vi "thermal_optical_camera_V2.vi"() -> ()   [LabVIEW 2025]
panel:
  out "file name out":string
  in  "File Path":string="C:\\Digambar\\Metal_thin_wall\\Optical_images\\Optical_images"
  in  "Stop (F)":bool
  in  "Acquisition Control:\nExposure Time [100, 3E7]":dbl=999.0 caption="Acquisition Control::Exposure Time" min=100.0 max=29999995.0
  in  "Analog Control:\nGain [0, 27]":dbl caption="Analog Control::Gain" min=0.0 max=27.045663671679687
  in  "Analog Control:\nBlack Level [-5, 10]":dbl caption="Analog Control::Black Level" min=-5.0000011920928955 max=10.000002384185791
  in  "Analog Control:\nGamma [0.25, 4.00]":dbl=0.800048828125 caption="Analog Control::Gamma" min=0.25 max=4.0 step=0.05
  out "Optical camera":T1(plugin-control)
  in  "optical capture interval (s)":dbl
  in  "thermal capture interval (s)":dbl
  out "Thermal camera":T1(plugin-control)
  out "IP address":string
  out "Output":string
  in  "Flag Button":bool
  in  "Stop Recording":bool
  in  "Stop Preview":bool
  in  "Focus":dbl(slide) scale=0.0..100.0
  in  "Record":bool
  # "Destination for Optical Images:"
  # "change folder names each time you run,\nso it saves data sets in dedicated folders:\nfolder1\nfolder2\nfolder3\netc..."
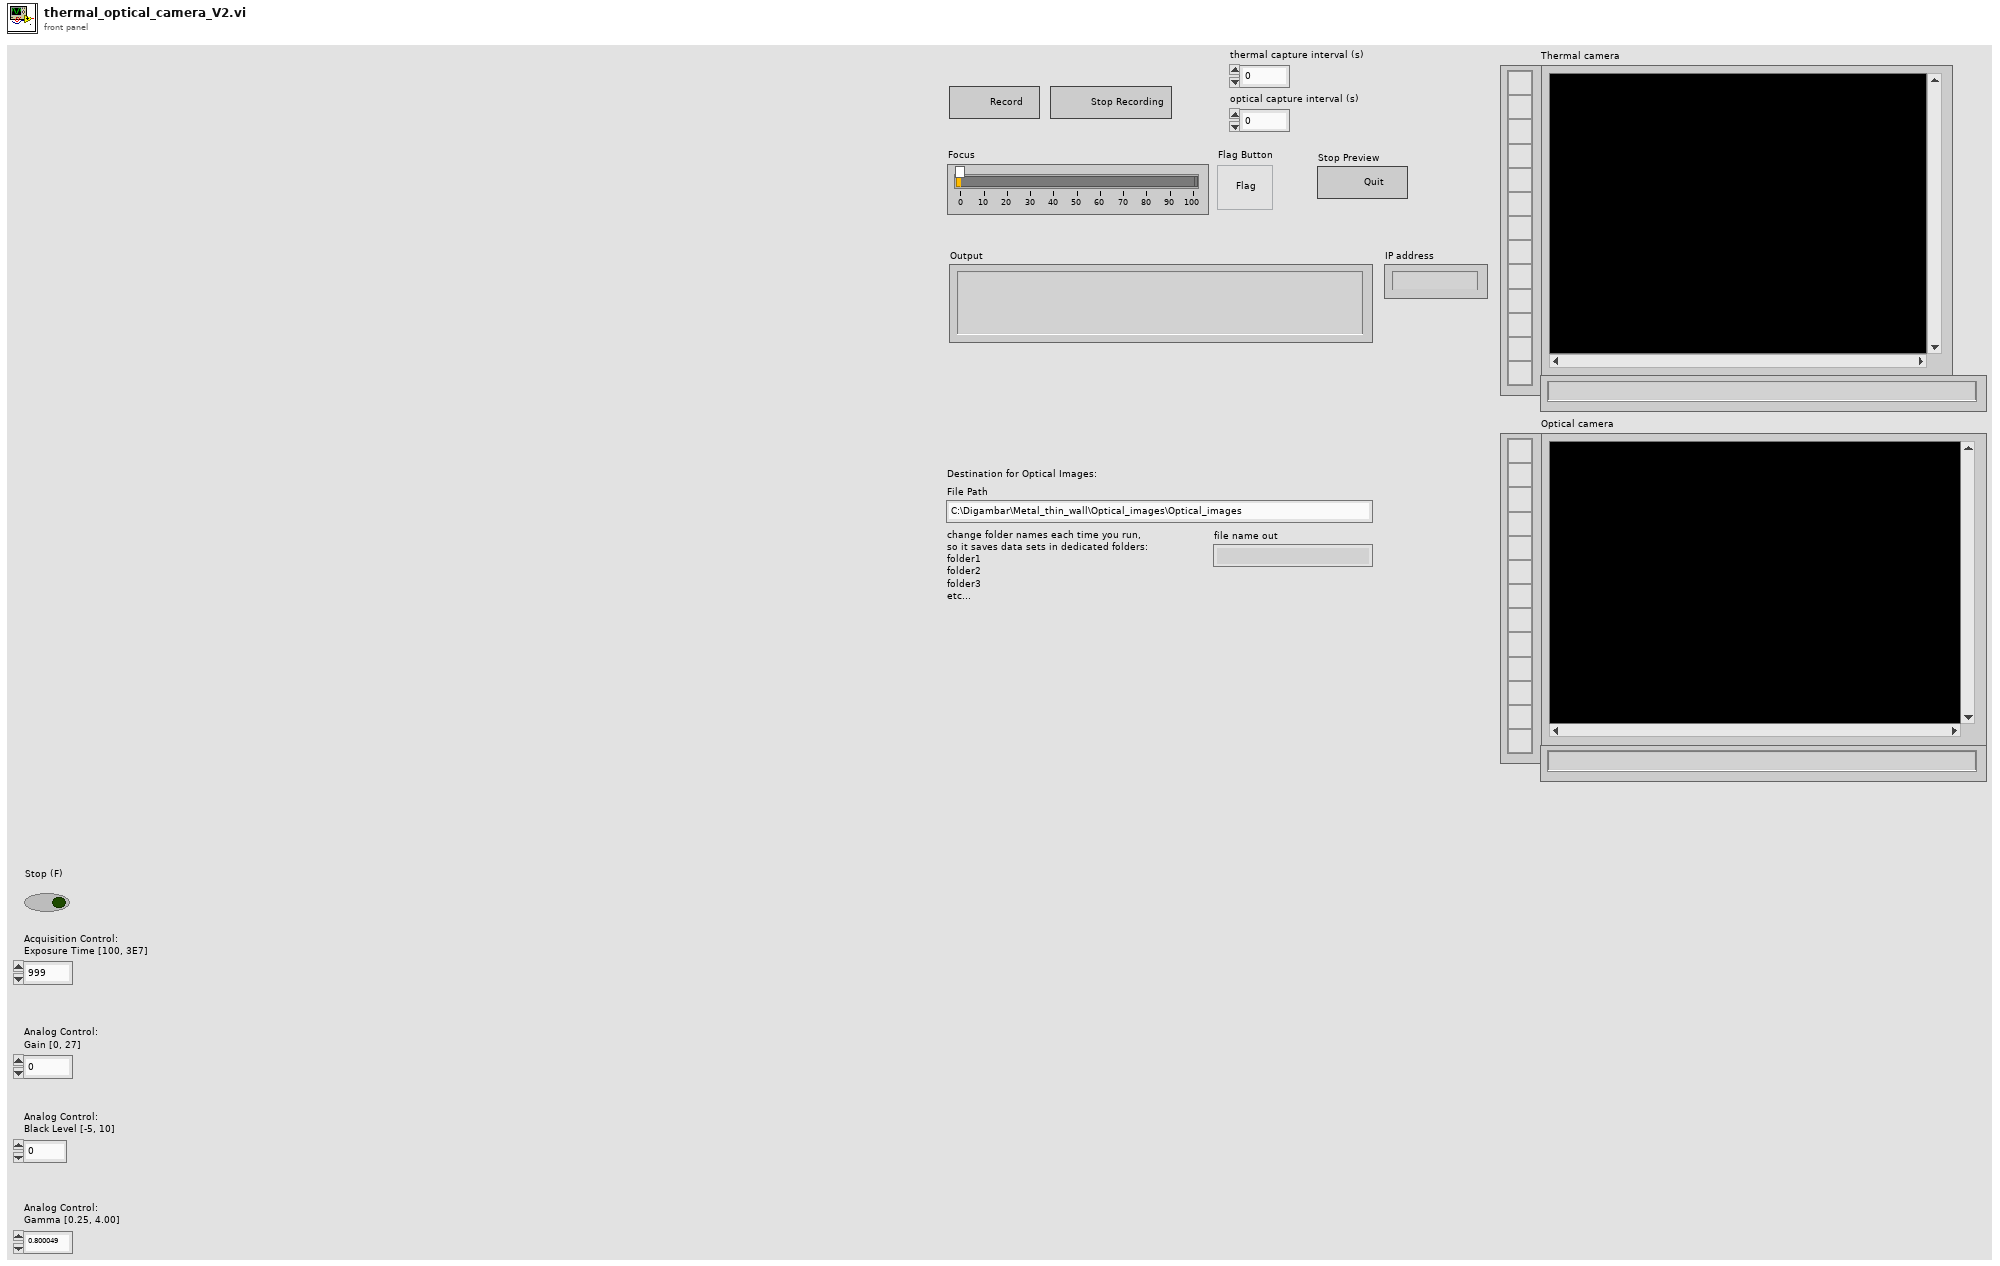
[diagram p1: front panel]
types:
  T1 = typedef "IMAQ Image.ctl" = refnum<image>
  T2 = enum16{"open", "replace", "create", "open or create", "replace or create", "replace or create with confirmation"}
  T3 = enum16{"big-endian, network order", "native, host order", "little-endian"}
  T4 = enum16{"Standard", "Buffered", "CRLF", "Immediate"}
  T5 = typedef "Image Type" = u32
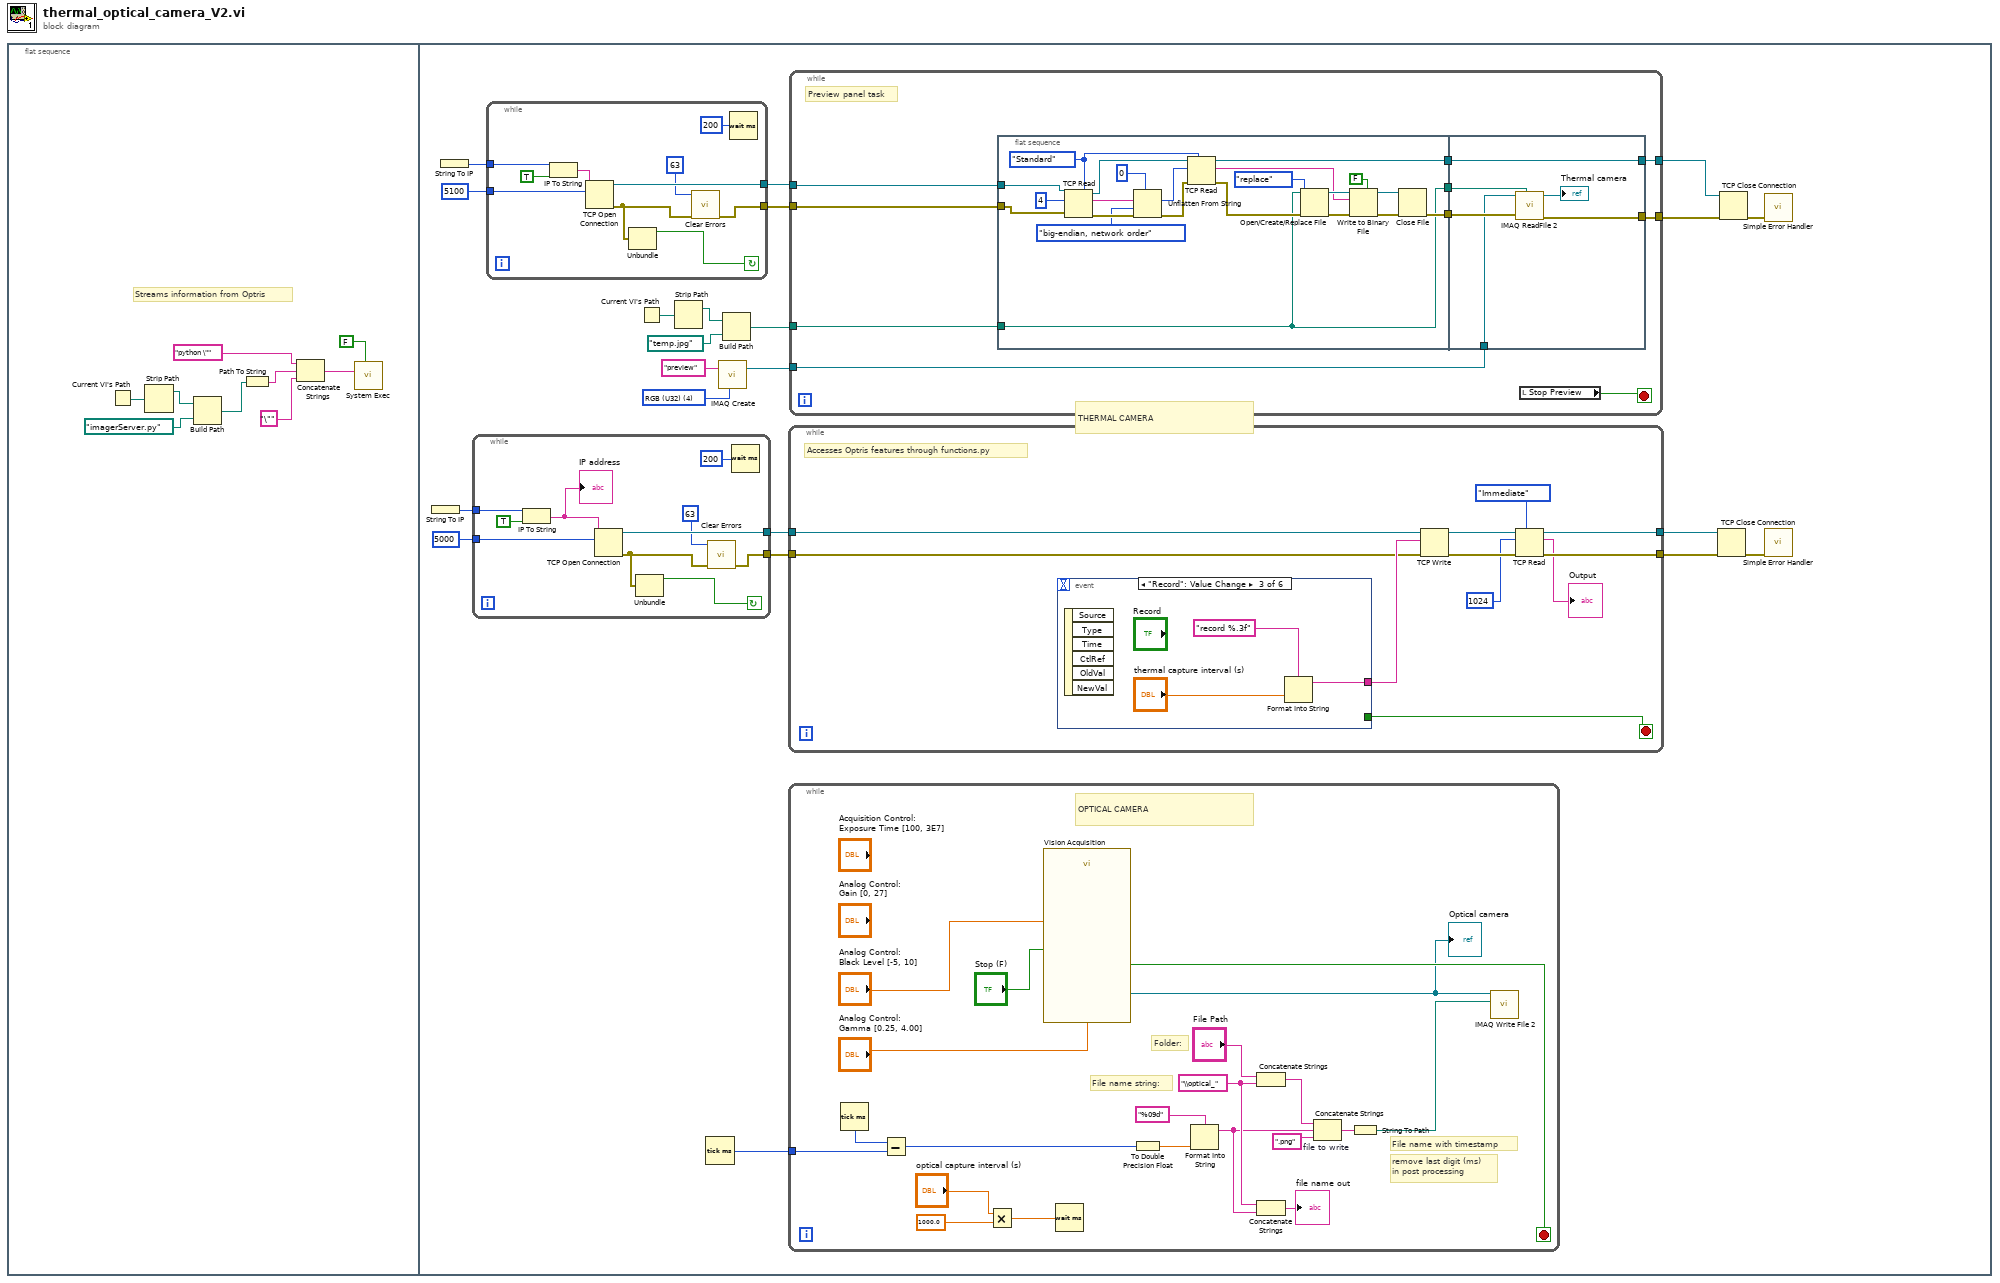
[diagram p0: block diagram]
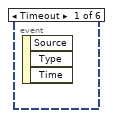
[diagram p2: hidden frame]
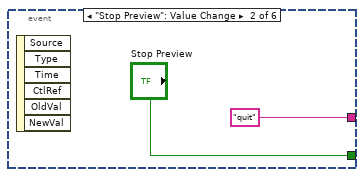
[diagram p3: hidden frame]
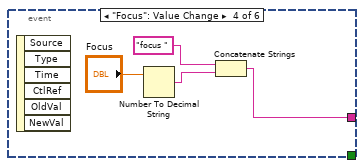
[diagram p4: hidden frame]
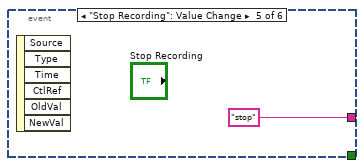
[diagram p5: hidden frame]
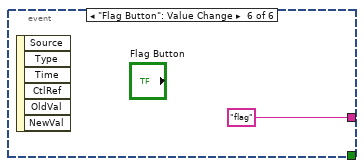
[diagram p6: hidden frame]
diagram:
  n1 = flat-sequence {
    frame #0 {
      # "Streams information from Optris"
      n2 = Current VI's Path() -> (path=w4:path)
      n3 = Strip Path(path=w4) -> (stripped path=w5:path)  [unwired: 1 out]
      n4 = Build Path(base path=w5, name or relative path=path "imagerServer.py") -> (appended path=w2:path)
      n5 = Path To String(path=w2) -> (string=w8:string)
      n6 = Concatenate Strings("python \"" ("string"), w8, "\"" ("string")) -> (w7:string)
      n7 = call <vilib>:"System Exec.vi"("wait until completion? (T)"=FALSE, "command line"=w7) -> ()  [unwired: 6 in, 4 out]
    }
    frame #1 {
      w19 = T5 4 items=["Grayscale (U8)", "Grayscale (I16)", "Grayscale (SGL)", "Complex (CSG)", "RGB (U32)", "HSL (U32)", "RGB (U64)", "Grayscale (U16)"] ("Image Type")
      # "THERMAL CAMERA"
      n8 = String To IP() -> (0:w16:u32)  [unwired: 1 in]
      n9 = String To IP() -> (0:w14:u32)  [unwired: 1 in]
      n10 = while {
        tunnel: [w66] -> w18
        tunnel: [w72] -> w17
        tunnel: w16 -> [w70]
        tunnel: u16 5000 ("remote port or service name") -> [w68]
        stop <- w63 continue-if-true
        n11 = IP To String(1:TRUE ("dot notation? (F)"), 2:w70) -> (0:w71:string)
        "IP address" <- w71
        n12 = TCP Open Connection(address=w71, remote port or service name=w68) -> (connection ID=w72:refnum<k5>, error out=w67:errorcluster)  [unwired: 3 in]
        n13 = Unbundle(w67) -> ("status"=w63:bool)  [unwired: 2 out]
        n14 = call <vilib>:"Clear Errors.vi"("error in (no error)"=w67, "specific error code to clear (0: all)"=63) -> ("error out"=w66:errorcluster)  [unwired: 4 in, 1 out]
        n15 = Wait (ms)(milliseconds to wait=u32 200) -> ()  [unwired: 1 out]
      }
      n16 = while {
        tunnel: w14 -> [w62]
        tunnel: [w56] -> w13
        tunnel: [w60] -> w12
        tunnel: u16 5100 ("remote port or service name") -> [w58]
        stop <- w53 continue-if-true
        n17 = IP To String(1:TRUE ("dot notation? (F)"), 2:w62) -> (0:w61:string)
        n18 = TCP Open Connection(address=w61, remote port or service name=w58) -> (connection ID=w60:refnum<k5>, error out=w57:errorcluster)  [unwired: 3 in]
        n19 = Unbundle(w57) -> ("status"=w53:bool)  [unwired: 2 out]
        n20 = call <vilib>:"Clear Errors.vi"("error in (no error)"=w57, "specific error code to clear (0: all)"=63) -> ("error out"=w56:errorcluster)  [unwired: 4 in, 1 out]
        n21 = Wait (ms)(milliseconds to wait=u32 200) -> ()  [unwired: 1 out]
      }
      n22 = Current VI's Path() -> (path=w30:path)
      n23 = Strip Path(path=w30) -> (stripped path=w31:path)  [unwired: 1 out]
      n24 = Tick Count (ms)() -> (millisecond timer value=w10:u32)
      n25 = call "IMAQ Create"("Image Name"="preview", "Image Type"=w19) -> ("New Image"=w26:T1)  [unwired: 3 in, 1 out]
      n26 = Build Path(base path=w31, name or relative path=path "temp.jpg") -> (appended path=w29:path)
      n27 = while {
        tunnel: [w120] -> w22
        tunnel: [w118] -> w23
        tunnel: w18 -> [w111]
        tunnel: w17 -> [w112]
        stop <- w113 stop-if-true
        # "Accesses Optris features through functions.py"
        n28 = event shown="[2] \"Record\": Value Change" {
          selector: _ -> [_ _ _ _ _ _]
          dyn-events: _ -> [_ _ _ _ _ _]
          timeout: _ -> [_ _ _ _ _ _]
          tunnel: [_ "quit" w126 w128 "stop" "flag"] -> w117
          tunnel: [_ "Stop Preview" _ _ _ _] -> w113
          event Timeout {
            n29 = event-data() -> ()  [unwired: 1 in, 3 out]
          }
          event "Stop Preview": Value Change {
            n30 = event-data() -> ()  [unwired: 1 in, 6 out]
          }
          event "Record": Value Change {
            n31 = event-data() -> ()  [unwired: 1 in, 6 out]
            n32 = Format Into String(format string="record %.3f", "thermal capture interval (s)") -> (resulting string=w126:string)  [unwired: 2 in, 1 out]
          }
          event "Focus": Value Change {
            n33 = event-data() -> ()  [unwired: 1 in, 6 out]
            n34 = Number To Decimal String(number="Focus") -> (decimal integer string=w130:string)  [unwired: 1 in]
            n35 = Concatenate Strings("focus ", w130) -> (w128:string)
          }
          event "Stop Recording": Value Change {
            n36 = event-data() -> ()  [unwired: 1 in, 6 out]
          }
          event "Flag Button": Value Change {
            n37 = event-data() -> ()  [unwired: 1 in, 6 out]
          }
        }
        n38 = TCP Write(connection ID=w112, data in=w117, error in (no error)=w111) -> (connection ID out=w119:refnum<k5>, error out=w121:errorcluster)  [unwired: 1 in, 1 out]
        n39 = TCP Read(connection ID=w119, bytes to read=1024, error in (no error)=w121, 7:T4."Immediate" ("mode (standard)")) -> (connection ID out=w118:refnum<k5>, data out=→"Output":string, error out=w120:errorcluster)  [unwired: 1 in]
      }
      n40 = while {
        tunnel: w10 -> [w40]
        stop <- w51 stop-if-true
        w37 = "\\optical_" ("string")
        # "OPTICAL CAMERA"
        # "remove last digit (ms)\nin post processing"
        # "File name with timestamp"
        # "Folder:"
        # "File name string:"
        n41 = Tick Count (ms)() -> (millisecond timer value=w41:u32)
        n42 = Subtract(x=w41, y=w40) -> (x-y=w32:u32)
        n43 = Multiply(x="optical capture interval (s)", y=1000.0) -> (x*y=w45:dbl)
        n44 = call "Vision Acquisition"("Analog Control::Black Level"="Analog Control:\nBlack Level [-5, 10]", "Analog Control::Gamma"="Analog Control:\nGamma [0.25, 4.00]", "Stop (F)"="Stop (F)") -> ("Image Out"=w50:T1, "Stopped"=w51:bool)  [unwired: 22 in, 1 out]
        "Optical camera" <- w50
        n45 = Wait (ms)(milliseconds to wait=w45) -> ()  [unwired: 1 out]
        n46 = To Double Precision Float(number=w32) -> (double precision float=w33:dbl)
        n47 = Format Into String(format string="%09d" ("time format string (%c)"), w33) -> (resulting string=w35:string)  [unwired: 2 in, 1 out]
        n48 = Concatenate Strings("File Path", w37) -> (w38:string)
        n49 = Concatenate Strings(w37, w35) -> (→"file name out":string)
        n50 = Concatenate Strings "file to write"(w38, w35, ".png" ("string")) -> (w47:string)
        n51 = String To Path(string=w47) -> (path=w43:path)
        n52 = call-poly "IMAQ Write File 2"("File Path"=w43, "Image"=w50) -> ()  [unwired: 8 in, 2 out]
      }
      n53 = while {
        tunnel: w26 -> [w77]
        tunnel: [w78] -> w27
        tunnel: [w82] -> w28
        tunnel: w29 -> [w80]
        tunnel: w13 -> [w75]
        tunnel: w12 -> [w74]
        stop <- w73 stop-if-true
        # "Preview panel task"
        n54 = flat-sequence {
          tunnel: w80 -> [w86]
          tunnel: [w88] -> w81
          tunnel: [w87] -> w79
          tunnel: [w86] -> w76
          tunnel: w75 -> [w84]
          tunnel: w74 -> [w83]
          tunnel: [w110] -> w82
          tunnel: w81 -> [w110]
          tunnel: w79 -> [w109]
          tunnel: [w108] -> w78
          tunnel: w77 -> [w107]
          tunnel: w76 -> [w106]
          frame #0 {
            w97 = T4."Standard" ("mode (standard)")
            n55 = TCP Read(connection ID=w83, bytes to read=4, error in (no error)=w84, 7:w97) -> (connection ID out=w100:refnum<k5>, data out=w85:string, error out=w103:errorcluster)  [unwired: 1 in]
            n56 = Unflatten From String(type=0, binary string=w85, byte order (0:big-endian, network order)=T3."big-endian, network order", error in (no error)=w103) -> (value=w98:i32, error out=w99:errorcluster)  [unwired: 1 in, 1 out]
            n57 = TCP Read(connection ID=w100, bytes to read=w98, error in (no error)=w99, 7:w97) -> (connection ID out=w88:refnum<k5>, data out=w93:string, error out=w95:errorcluster)  [unwired: 1 in]
            n58 = Open/Create/Replace File(file path (use dialog)=w86, error in=w95, operation (0:open)=T2."replace") -> (refnum out=w94:refnum<file>, error out=w91:errorcluster)  [unwired: 3 in, 1 out]
            n59 = Write to Binary File(file (use dialog)=w94, data=w93, error in=w91, 5:FALSE ("prepend array or string size? (T)")) -> (refnum out=w89:refnum<file>, error out=w90:errorcluster)  [unwired: 2 in, 1 out]
            n60 = Close File(refnum=w89, error in=w90) -> (error out=w87:errorcluster)  [unwired: 1 out]
          }
          frame #1 {
            n61 = call "IMAQ ReadFile 2"("File Path"=w106, "error in (no error)"=w109, "Image"=w107) -> ("error out"=w108:errorcluster, "Image Out"=→"Thermal camera":T1)  [unwired: 4 in, 3 out]
          }
        }
        n62 = local read "Stop Preview"() -> (w73:bool)
      }
      n63 = TCP Close Connection(connection ID=w23, error in (no error)=w22) -> (error out=w24:errorcluster)  [unwired: 1 in, 1 out]
      n64 = TCP Close Connection(connection ID=w28, error in (no error)=w27) -> (error out=w25:errorcluster)  [unwired: 1 in, 1 out]
      n65 = call <vilib>:"Simple Error Handler.vi"("error in (no error)"=w25) -> ()  [unwired: 4 in, 5 out]
      n66 = call <vilib>:"Simple Error Handler.vi"("error in (no error)"=w24) -> ()  [unwired: 4 in, 5 out]
    }
  }
